vi "test String to I16_1.vi"(11 "Test Case In":refnum<class "test Electronic Datasheet.lvclass">) -> (0 "error out":errorcluster, 3 "Test Case Out":refnum<class "test Electronic Datasheet.lvclass">)   [LabVIEW 2024, in "Test Utilities.lvclass"]
uses:
  Test Utilities.lvclass
  Test Utilities.lvclass/Test Utilities.ctl
  EDS-File-Viewer/Tests/source/test Electronic Datasheet/test Electronic Datasheet.lvclass
  <vilib>/Astemes/LUnit/Test Case.lvclass
  source/CANopen.lvlib
panel:
  out "I16":i16
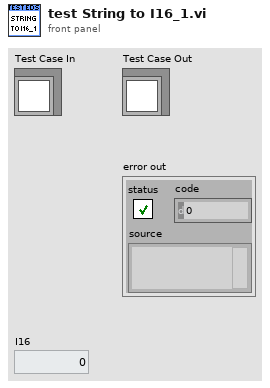
[diagram p1: front panel]
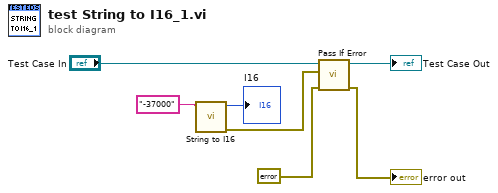
[diagram p0: block diagram]
diagram:
  n1 = call "String to I16.vi"("Integer String"="-37000" ("String")) -> ("error out"=w3:errorcluster, "I16"=→"I16":i16)  [unwired: 9 in]
  n2 = call <vilib>:"Pass If Error.vi"("error in (no error)"=errorcluster {"status"=FALSE, "code"=0, "source"=""}, "Assert error"=w3, "LUnit Test Case In"="Test Case In") -> ("error out"=→"error out":errorcluster, "LUnit Test Case Out"=→"Test Case Out":refnum<class "test Electronic Datasheet.lvclass">)  [unwired: 7 in]
